vi "CRYCalc Directivity LW.vi"(7 "Direct_weight":bool caption="Weighting", 8 "weight":dbl, 9 "Degree":dbl, 10 "In L(f)":dbl, 11 "Y ref":dbl=1.0) -> (1 "L(f)*W(deg)":dbl)   [LabVIEW 2013]
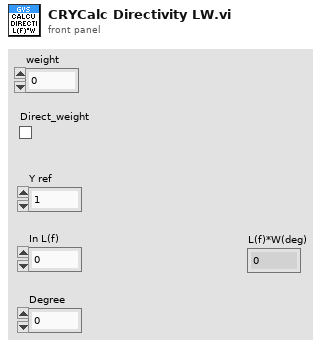
[diagram p1: front panel]
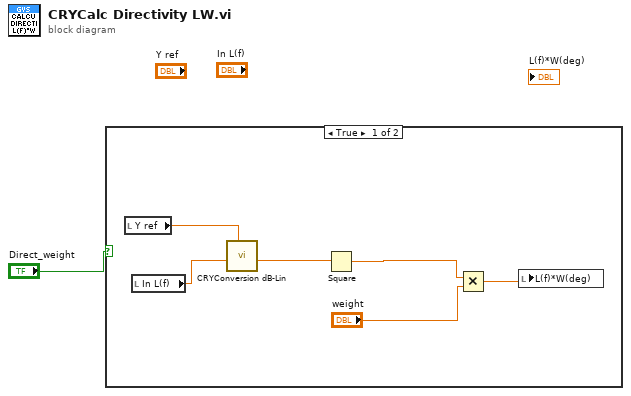
[diagram p0: block diagram]
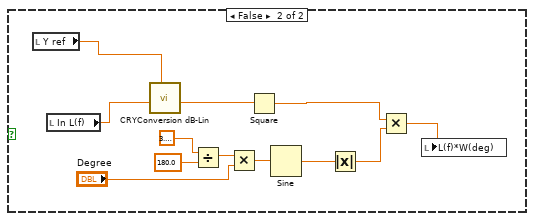
[diagram p2: hidden frame]
diagram:
  n1 = case shown="True" "Direct_weight" {
    frame True {
      n2 = local read "Y ref"() -> (w4:dbl)
      n3 = local read "In L(f)"() -> (w3:dbl)
      n4 = call "CRYConversion dB-Lin.vi"("dB ref."=w4, "Log In"=w3) -> ("Lin Out"=w7:dbl)  [unwired: 4 in, 3 out]
      n5 = Square(x=w7) -> (x^2=w6:dbl)
      n6 = Multiply(x=w6, y="weight") -> (x*y=w2:dbl)
      n7 = local write "L(f)*W(deg)"(w2) -> ()
    }
    frame False {
      n8 = local read "Y ref"() -> (w10:dbl)
      n9 = local read "In L(f)"() -> (w9:dbl)
      n10 = call "CRYConversion dB-Lin.vi"("dB ref."=w10, "Log In"=w9) -> ("Lin Out"=w12:dbl)  [unwired: 4 in, 3 out]
      n11 = Divide(x=3.141592653589793, y=180.0) -> (x/y=w16:dbl)
      n12 = Multiply(x=w16, y="Degree") -> (x*y=w17:dbl)
      n13 = Square(x=w12) -> (x^2=w11:dbl)
      n14 = Sine(x=w17) -> (sin(x)=w14:dbl)
      n15 = Absolute Value(x=w14) -> (abs(x)=w13:dbl)
      n16 = Multiply(x=w11, y=w13) -> (x*y=w8:dbl)
      n17 = local write "L(f)*W(deg)"(w8) -> ()
    }
  }
